vi "Fixed Counter with Semaphore.vi"() -> ()   [LabVIEW 2012]
panel:
  out "Running Total":i32
  in  "Stop Button":bool
  out "Loop Count Difference":i32
  out "Loop Count 2":i32
  out "Loop Count 1":i32
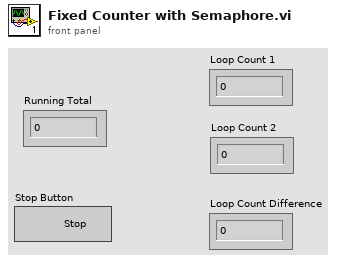
[diagram p1: front panel]
types:
  T1 = typedef "Semaphore RefNum" = refnum<k1>
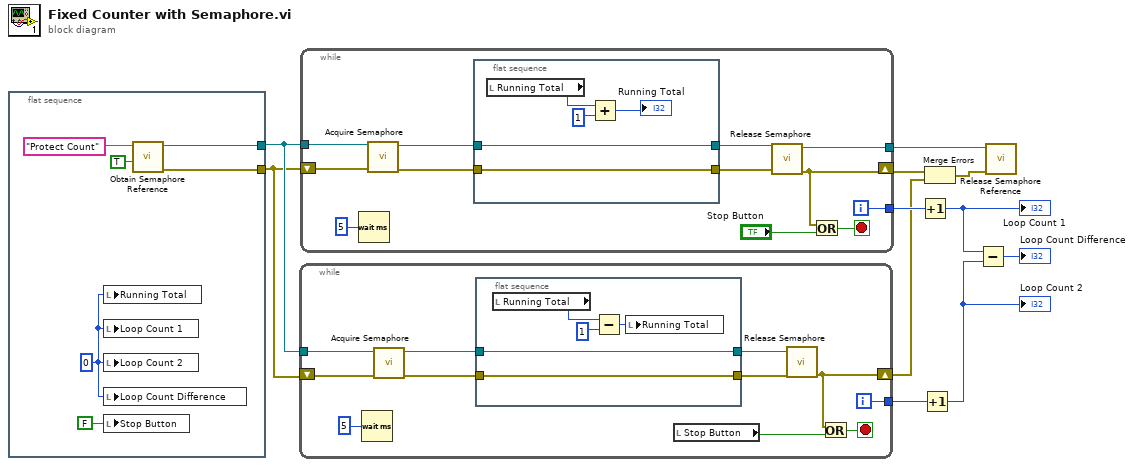
[diagram p0: block diagram]
diagram:
  n1 = flat-sequence {
    tunnel: [w15] -> w5
    tunnel: [w14] -> w6
    frame #0 {
      w12 = 0 ("Running Total")
      n2 = local write "Running Total"(w12) -> ()
      n3 = local write "Loop Count 1"(w12) -> ()
      n4 = local write "Loop Count 2"(w12) -> ()
      n5 = local write "Loop Count Difference"(w12) -> ()
      n6 = local write "Stop Button"(FALSE ("Stop Button")) -> ()
      n7 = call <vilib>:"Obtain Semaphore Reference.vi"("create if not found (T)"=TRUE, "name (unnamed)"="Protect Count") -> ("error out"=w15:errorcluster, "semaphore"=w14:T1)  [unwired: 3 in, 1 out]
    }
  }
  n8 = while {
    tunnel: [w27] -> w10
    tunnel: w6 -> [w26]
    shift-right: [w18] -> w1
    shift-left: w5 -> [w25]
    i -> [w27]
    stop <- w21 stop-if-true
    n9 = Wait (ms)(milliseconds to wait=u32 5) -> ()  [unwired: 1 out]
    n10 = call <vilib>:"Acquire Semaphore.vi"("error in (no error)"=w25, "semaphore"=w26) -> ("error out"=w24:errorcluster, "semaphore out"=w23:T1)  [unwired: 3 in, 1 out]
    n11 = flat-sequence {
      tunnel: w24 -> [w29]
      tunnel: w23 -> [w30]
      tunnel: [w30] -> w22
      tunnel: [w29] -> w19
      frame #0 {
        n12 = local read "Running Total"() -> (w33:i32)
        n13 = Subtract(x=w33, y=1 ("x")) -> (x-y=w31:i32)
        n14 = local write "Running Total"(w31) -> ()
      }
    }
    n15 = local read "Stop Button"() -> (w20:bool)
    n16 = call <vilib>:"Release Semaphore.vi"("error in (no error)"=w19, "semaphore"=w22) -> ("error out"=w18:errorcluster)  [unwired: 4 in, 1 out]
    n17 = Or(x=w18, y=w20) -> (x .or. y?=w21:bool)
  }
  n18 = while {
    tunnel: [w43] -> w11
    tunnel: w6 -> [w42]
    tunnel: [w36] -> w4
    shift-right: [w34] -> w3
    shift-left: w5 -> [w41]
    i -> [w43]
    stop <- w35 stop-if-true
    n19 = Wait (ms)(milliseconds to wait=u32 5) -> ()  [unwired: 1 out]
    n20 = call <vilib>:"Acquire Semaphore.vi"("error in (no error)"=w41, "semaphore"=w42) -> ("error out"=w40:errorcluster, "semaphore out"=w38:T1)  [unwired: 3 in, 1 out]
    n21 = flat-sequence {
      tunnel: w40 -> [w47]
      tunnel: [w47] -> w39
      tunnel: w38 -> [w46]
      tunnel: [w46] -> w37
      frame #0 {
        n22 = local read "Running Total"() -> (w49:i32)
        n23 = Add(x=w49, y=1 ("x")) -> (x+y=→"Running Total":i32)
      }
    }
    n24 = call <vilib>:"Release Semaphore.vi"("error in (no error)"=w39, "semaphore"=w37) -> ("error out"=w34:errorcluster, "semaphore out"=w36:T1)  [unwired: 4 in]
    n25 = Or(x=w34, y="Stop Button") -> (x .or. y?=w35:bool)
  }
  n26 = Increment(x=w11) -> (x+1=w9:i32)
  "Loop Count 1" <- w9
  n27 = Increment(x=w10) -> (x+1=w8:i32)
  "Loop Count 2" <- w8
  n28 = Merge Errors(w3, w1) -> (w2:errorcluster)
  n29 = Subtract(x=w9, y=w8) -> (x-y=→"Loop Count Difference":i32)
  n30 = call <vilib>:"Release Semaphore Reference.vi"("error in (no error)"=w2, "semaphore"=w4) -> ()  [unwired: 8 in, 2 out]
